vi "ConvertMatlabDataValueToBoolean.vi"(11 "Data Value":variant) -> (3 "Boolean":bool)   [LabVIEW 2017]
uses:
  <vilib>/Utility/Data Type/Type Definitions/Data Type.ctl
  <vilib>/Utility/Data Type/NI_Data Type.lvlib
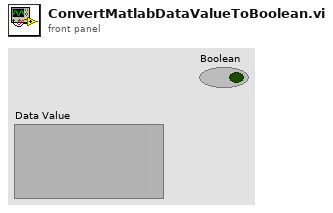
[diagram p1: front panel]
types:
  T1 = typedef "NI_Data Type.lvlib/Data Type.ctl" = enum8{"Invalid Type", "Void", "I8", "I16", "I32", "I64", "U8", "U16", "U32", "U64", "Single Float", "Double Float", "Extended Float", "Single Complex", "Double Complex", "Extended Complex", "Enum U8", "Enum U16", "Enum U32", "Enum U64", "Single Float With Unit", "Double Float With Unit", "Extended Float With Unit", "Single Complex with Unit", "Double Complex with Unit", "Extended Complex with Unit", "Boolean", "String", "Path", "Picture", "Tag", "Array", "Cluster", "Variant", "LV Variant", "Waveform", "Timestamp", "Digital Waveform", "Digital Data", "ExpressData", "Refnum", "External Data", "VI", "Poly VI", "LabVIEW Class Instance", "Fixed Point"}
  T2 = typedef "MatlabDataType.ctl" = enum16{"NotAMatlabType", "Real", "Complex", "String", "Boolean"}
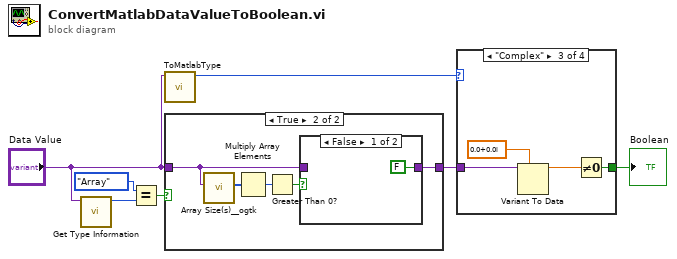
[diagram p0: block diagram]
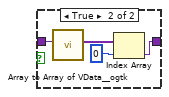
[diagram p3: hidden frame]
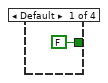
[diagram p4: hidden frame]
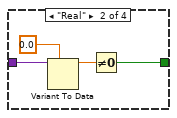
[diagram p5: hidden frame]
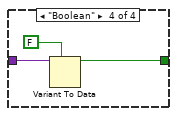
[diagram p6: hidden frame]
diagram:
  n1 = call <vilib>:"Get Type Information.vi"("Variant"="Data Value") -> ("Type"=w5:T1)  [unwired: 6 in, 4 out]
  n2 = Equal?(x=Data_Type."Array" ("Type"), y=w5) -> (x = y?=w6:bool)
  n3 = call "ToMatlabType.vi"("Value"="Data Value") -> ("MatlabType"=w1:T2)  [unwired: 6 in, 4 out]
  n4 = case shown="True" w6 {
    tunnel: "Data Value" -> [w8 w12]
    tunnel: [w8 w13] -> w7
    frame False {
    }
    frame True {
      n5 = call <userlib>:"Array Size(s)__ogtk.vi"("Array"=w12) -> ("Size(s)"=w11:u32[])  [unwired: 8 in, 2 out]
      n6 = Multiply Array Elements(1:w11) -> (0:w10:u32)
      n7 = Greater Than 0?(x=w10) -> (x > 0?=w9:bool)
      n8 = case shown="False" w9 {
        tunnel: [FALSE w16] -> w13
        tunnel: w12 -> [_ w15]
        frame False {
        }
        frame True {
          n9 = call <userlib>:"Array to Array of VData__ogtk.vi"("MultiD Array"=w15) -> ("1D Array of Variants"=w18:variant[])  [unwired: 9 in, 1 out]
          n10 = Index Array(array=w18, index=0) -> (element=w16:variant)
        }
      }
    }
  }
  n11 = case shown="\"Complex\"" w1 {
    tunnel: w7 -> [_ w23 w27 w29]
    tunnel: [FALSE w20 w24 w28] -> w3
    frame Default {
    }
    frame "Real" {
      n12 = Variant To Data(type=0.0, Variant=w23) -> (data=w21:dbl)  [unwired: 1 in, 1 out]
      n13 = Not Equal To 0?(x=w21) -> (x != 0?=w20:bool)
    }
    frame "Complex" {
      n14 = Variant To Data(type=cdb 0.0+0.0i, Variant=w27) -> (data=w25:cdb)  [unwired: 1 in, 1 out]
      n15 = Not Equal To 0?(x=w25) -> (x != 0?=w24:bool)
    }
    frame "Boolean" {
      n16 = Variant To Data(type=FALSE, Variant=w29) -> (data=w28:bool)  [unwired: 1 in, 1 out]
    }
  }
  "Boolean" <- w3
